vi "Leak check Protokoll_Kopf.vi"(11 "Externer Fehler":bool) -> ()   [LabVIEW 2020, in "EPA 1065.lvlib" / "Dichtheitstest 1065-345.lvlib"]
uses:
  Dichtheitstest 1065-345.lvlib
  Aktion Protokolldaten_Leak check.ctl
  Sprachverwaltung/FGV Aktion Tabelle zerlegen.ctl
  Funktionstasten/Funktionstasten-Aktion.ctl
  Seiten/System Einstellungen V2/Aktioen FGV System Konstanten.ctl
  Aktion Leak Daten.ctl
  PDF_Interface/PDF Protokoll Standard Kopf Optionen.ctl
  Sprachverwaltung/Sprachverwaltung.lvlib
  Funktionstasten/Funktionstasten.lvlib
  Seiten/System Einstellungen V2/System Einstellungen V2.lvlib
  Linearisierung V2/Protokoll/Protokoll.lvlib
  PDF_Interface/PDF Interface.lvlib
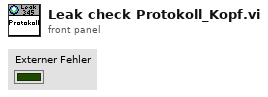
[diagram p1: front panel]
types:
  T1 = typedef "PDF Interface.lvlib/PDF Protokoll Standard Kopf Optionen.ctl" = cluster{"Analysator":bool, "FT-IR Rezept":bool, "Gasteiler":bool, "Gas Komponente":bool, "Gas Flasche":bool, "LIN Protokoll":bool, "Operator":bool}
  T2 = typedef "EPA 1065.lvlib/Dichtheitstest 1065-345.lvlib/Aktion Leak Daten.ctl" = enum16{"lesen", "laden", "speichern", "Volumen", "berechnen", "Leak check aktiv", "Leak Zustand", "Pfad", "Pfad speichern"}
  T3 = typedef "System Einstellungen V2.lvlib/Aktioen FGV System Konstanten.ctl" = enum16{"lesen", "laden", "speichern", "Sprache"}
  T4 = typedef "Funktionstasten.lvlib/Funktionstasten-Aktion.ctl" = enum16{"Initialisieren", "Zustand setzen", "Taste gedrückt", "Fehler speichern", "Lesen", "Manuell", "Remote", "Bitparallel", "Samplepoint", "Zeit Prüfen", "reset Umschalten"}
  T5 = typedef "Sprachverwaltung.lvlib/FGV Aktion Tabelle zerlegen.ctl" = enum16{"laden", "vereinzeln", "speichern"}
  T6 = typedef "EPA 1065.lvlib/Dichtheitstest 1065-345.lvlib/Aktion Protokolldaten_Leak check.ctl" = enum16{"lesen", "Zeitstempel", "Bearbeiter", "Daten", "Auswertung", "löschen"}
  T7 = typedef "EPA 1065.lvlib/Dichtheitstest 1065-345.lvlib/Leak Daten.ctl" = cluster{"Gesamtes Volumen":sgl, "p 1":sgl, "p 2":sgl, "T 1":sgl, "T 2":sgl, "t 1":timestamp, "t 2":timestamp, "Ergebnis mol/s":sgl, "Grenze mol/s":sgl, "Leak in %":sgl, "Ergebnis mbar":sgl, "Grenze mbar":sgl}
  T8 = cluster{"Modell":string, "ProjektNummer":string, "Software Version":string, "Seriennummer":string}
  T9 = typedef "EPA 1065.lvlib/Dichtheitstest 1065-345.lvlib/Gesamtvolumen.ctl" = cluster{"FAS":sgl, "d von HL zu VFS":sgl, "l von HL zu VFS":sgl, "VFS":sgl, "d von HL zu SP":sgl, "l von HL zu SP":sgl, "Heizleitung zum VFS":bool, "VFS a":bool, "Heizleitung zur Entnahmestelle":bool, "Gesamtes Volumen":sgl, "LeakValve":u16, "Einheit":enum16{"mol/s", "mbar"}}
  T10 = typedef "EPA 1065.lvlib/Dichtheitstest 1065-345.lvlib/Leak Protokoll Einstellungen.ctl" = cluster{"Bearbeiter:":string, "Pfad:":path, "Textname:":string, "Analysator":T11}
  T11 = typedef "System Einstellungen V2.lvlib/Analysatoren.ctl" = string
  T12 = typedef "String - Ausgabefeld.ctl" = string
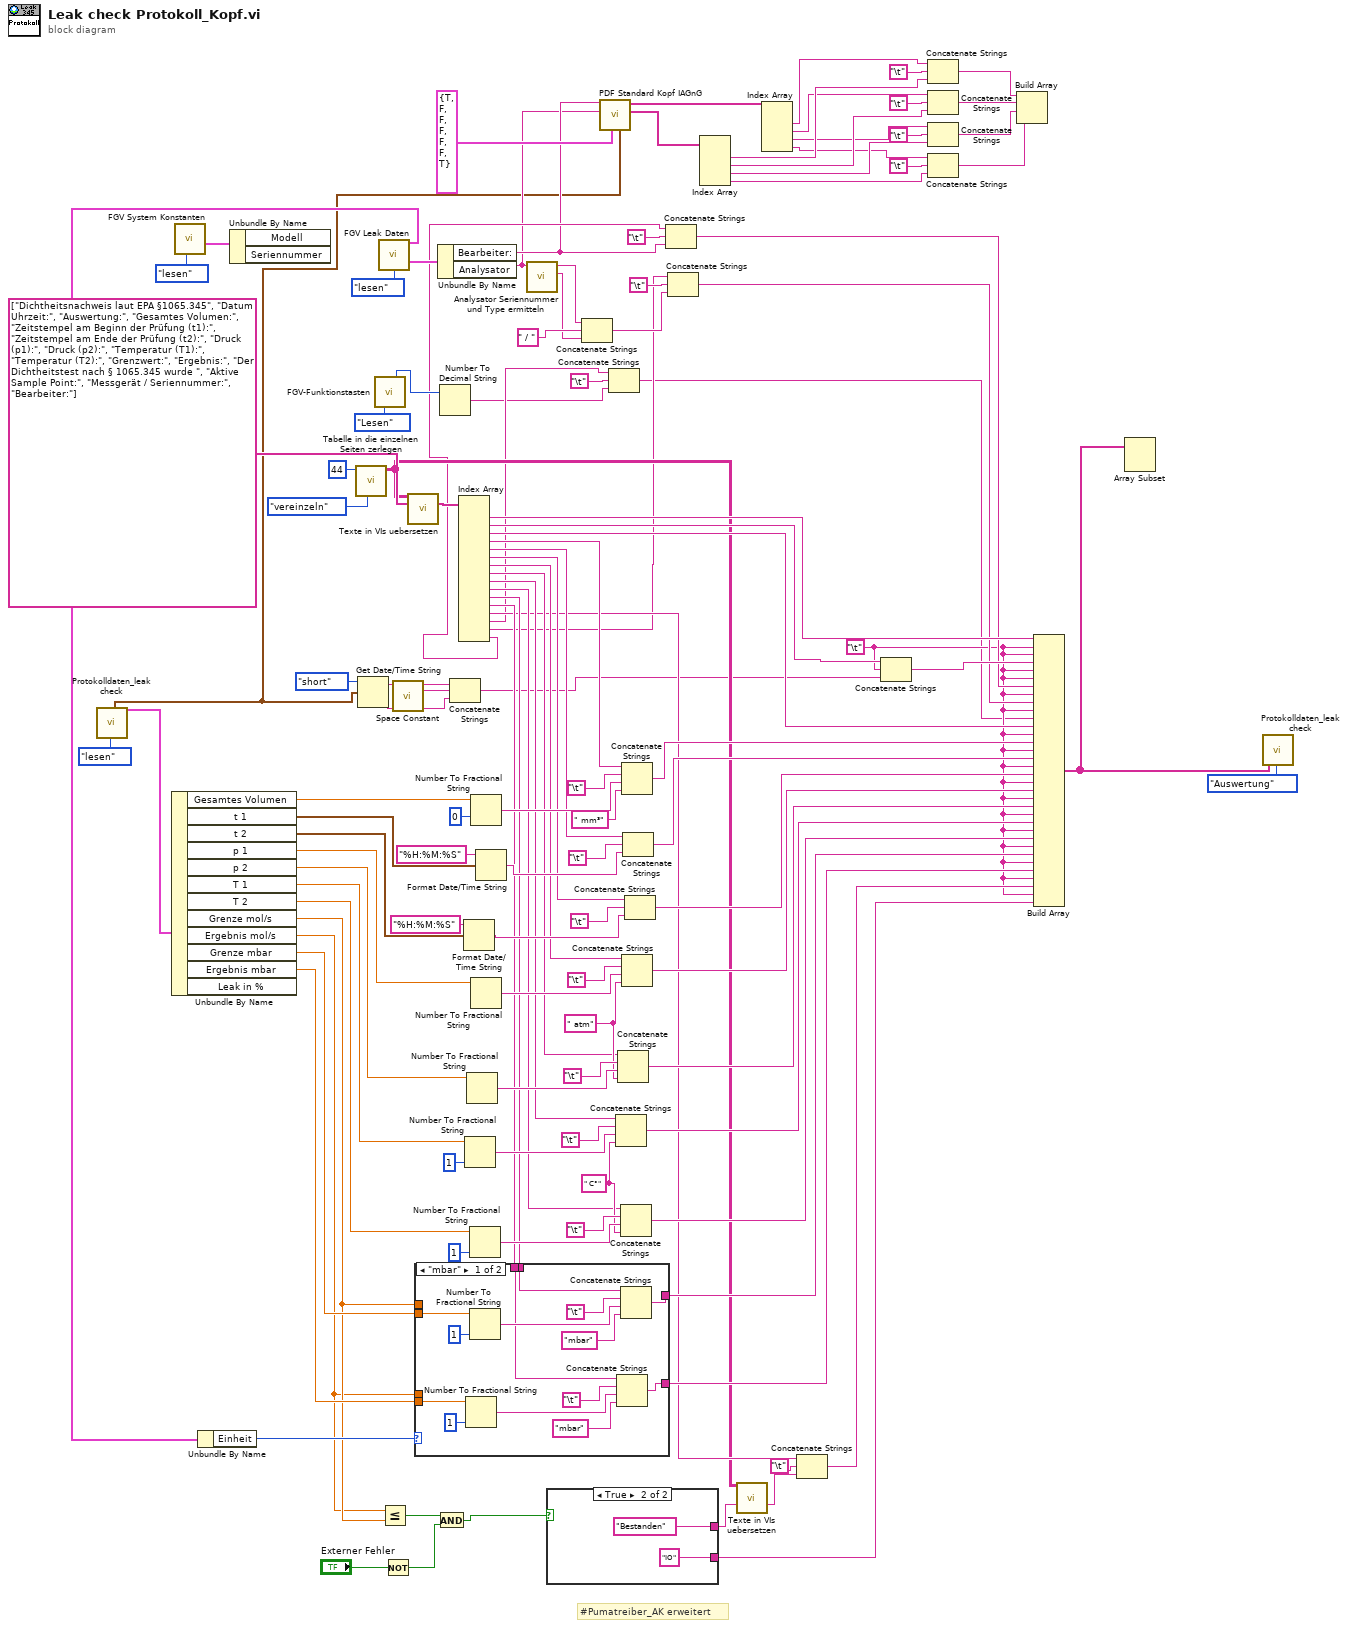
[diagram p0: block diagram]
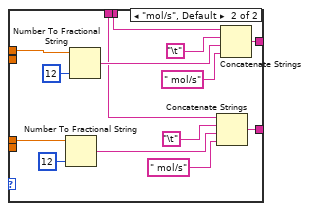
[diagram p2: hidden frame]
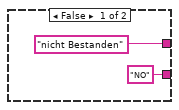
[diagram p3: hidden frame]
diagram:
  w42 = "\t"
  w99 = " C°"
  w100 = " atm"
  # "#Pumatreiber_AK erweitert"
  n1 = call "Protokolldaten_leak check.vi"("Aktion"=Aktion_Protokolldaten_Leak_check."lesen") -> ("Start"=w1:timestamp, "Daten"=w39:T7)  [unwired: 23 in, 2 out]
  n2 = Unbundle By Name(w39) -> ("Gesamtes Volumen"=w38:sgl, "t 1"=w37:timestamp, "t 2"=w36:timestamp, "p 1"=w35:sgl, "p 2"=w34:sgl, "T 1"=w33:sgl, "T 2"=w32:sgl, "Grenze mol/s"=w27:sgl, "Ergebnis mol/s"=w26:sgl, "Grenze mbar"=w28:sgl, "Ergebnis mbar"=w29:sgl)  [unwired: 1 out]
  n3 = call "FGV System Konstanten.vi"("Aktionen"=Aktioen_FGV_System_Konstanten."lesen") -> ("Cluster out"=w53:T8)  [unwired: 6 in, 4 out]
  n4 = Unbundle By Name(w53) -> ()  [unwired: 2 out]
  n5 = call "Tabelle in die einzelnen Seiten zerlegen.vi"("Aktion"=FGV_Aktion_Tabelle_zerlegen."vereinzeln", "Index (Seite)"=44) -> ("Sprachliste"=w64:string[][])  [unwired: 7 in, 2 out]
  n6 = Get Date/Time String(date format (0)=enum16{"short", "long", "abbreviated"}."short" ("Datumsformat (0)"), seconds (now)=w1) -> (date string=w122:string, time string=w120:string)  [unwired: 1 in]
  n7 = call "FGV-Funktionstasten.vi"("Aktion"=Funktionstasten-Aktion."Lesen") -> ("Samplepoint"=w56:u16)  [unwired: 7 in, 7 out]
  n8 = call "FGV Leak Daten.vi"("Aktion"=Aktion_Leak_Daten."lesen") -> ("Gesamtvolumen"=w31:T9, "Leak Protokoll"=w47:T10)  [unwired: 10 in, 3 out]
  n9 = Unbundle By Name(w31) -> ("Einheit"=w30:enum16{"mol/s", "mbar"})
  n10 = Less Or Equal?(x=w26, y=w27) -> (x <= y?=w84:bool)
  n11 = Not(x="Externer Fehler") -> (.not. x?=w83:bool)
  n12 = call <vilib>:"Space Constant.vi"() -> ("String"=w121:string)
  n13 = call "Texte in VIs uebersetzen.vi"("Sprachliste"=w64, "String-Array zum Übersetzen"=string[] ["Dichtheitsnachweis laut EPA §1065.345", "Datum Uhrzeit:", "Auswertung:", "Gesamtes Volumen:", "Zeitstempel am Beginn der Prüfung (t1):", "Zeitstempel am Ende der Prüfung (t2):", "Druck (p1):", "Druck (p2):", "Temperatur (T1):", "Temperatur (T2):", "Grenzwert:", "Ergebnis:", "Der Dichtheitstest nach § 1065.345 wurde ", "Aktive Sample Point:", "Messgerät / Seriennummer:", "Bearbeiter:"]) -> ("String-Array zum Übersetzen"=w80:string[])  [unwired: 9 in, 4 out]
  n14 = And(x=w84, y=w83) -> (x .and. y?=w86:bool)
  n15 = Unbundle By Name(w47) -> ("Bearbeiter:"=w22:string, "Analysator"=w21:T11)
  n16 = Number To Decimal String(number=w56) -> (decimal integer string=w55:string)  [unwired: 1 in]
  n17 = Concatenate Strings(w122, w121, w120) -> (w60:string)
  n18 = Index Array(array=w80) -> (element #1=w79:string, element #2=w78:string, element #3=w77:string, element #4=w76:string, element #5=w75:string, element #6=w74:string, element #7=w73:string, element #8=w72:string, element #9=w71:string, element #10=w70:string, element #11=w69:string, element #12=w68:string, element #13=w67:string, element #14=w57:string, element #15=w49:string, element #16=w45:string)  [unwired: 16 in]
  n19 = case shown="\"mbar\"" w30 {
    tunnel: [w132 w146] -> w98
    tunnel: [w131 w145] -> w97
    tunnel: w69 -> [w128 w142]
    tunnel: w68 -> [w127 w141]
    tunnel: w27 -> [_ w140]
    tunnel: w26 -> [_ w139]
    tunnel: w28 -> [w126 _]
    tunnel: w29 -> [w125 _]
    frame "mbar" {
      n20 = Number To Fractional String(number=w125, precision (6)=i16 1 ("Genauigkeit (6)")) -> (F-format string=w133:string)  [unwired: 2 in]
      n21 = Number To Fractional String(number=w126, precision (6)=i16 1 ("Genauigkeit (6)")) -> (F-format string=w138:string)  [unwired: 2 in]
      n22 = Concatenate Strings(w127, "\t", w133, "mbar") -> (w131:string)
      n23 = Concatenate Strings(w128, "\t", w138, "mbar") -> (w132:string)
    }
    frame "mol/s", Default {
      n24 = Number To Fractional String(number=w139, precision (6)=i16 12 ("Genauigkeit (6)")) -> (F-format string=w147:string)  [unwired: 2 in]
      n25 = Number To Fractional String(number=w140, precision (6)=i16 12 ("Genauigkeit (6)")) -> (F-format string=w152:string)  [unwired: 2 in]
      n26 = Concatenate Strings(w141, "\t", w147, " mol/s") -> (w145:string)
      n27 = Concatenate Strings(w142, "\t", w152, " mol/s") -> (w146:string)
    }
  }
  n28 = Format Date/Time String(time format string (%c)="%H:%M:%S" ("Zeitformatierungs-String (%c)"), seconds (now)=w36) -> (date/time string=w88:string)  [unwired: 1 in]
  n29 = Number To Fractional String(number=w33, precision (6)=i16 1 ("Genauigkeit (6)")) -> (F-format string=w108:string)  [unwired: 2 in]
  n30 = Number To Fractional String(number=w34) -> (F-format string=w109:string)  [unwired: 3 in]
  n31 = Number To Fractional String(number=w32, precision (6)=i16 1 ("Genauigkeit (6)")) -> (F-format string=w105:string)  [unwired: 2 in]
  n32 = Number To Fractional String(number=w38, precision (6)=i16 0 ("Genauigkeit (6)")) -> (F-format string=w118:string)  [unwired: 2 in]
  n33 = Number To Fractional String(number=w35) -> (F-format string=w116:string)  [unwired: 3 in]
  n34 = Format Date/Time String(time format string (%c)="%H:%M:%S" ("Zeitformatierungs-String (%c)"), seconds (now)=w37) -> (date/time string=w90:string)  [unwired: 1 in]
  n35 = call "Analysator Seriennummer und Type ermitteln.vi"("Analysator"=w21) -> ("Type"=w24:string, "Name für Protokoll"=w25:string)  [unwired: 8 in, 1 out]
  n36 = case shown="True" w86 {
    tunnel: ["nicht Bestanden" ("Element") "Bestanden" ("Element")] -> w66
    tunnel: ["NO" ("Element") "IO" ("Element")] -> w40
    frame False {
    }
    frame True {
    }
  }
  n37 = Concatenate Strings(w25, " / ", w24) -> (w50:string)
  n38 = call "PDF Standard Kopf IAGnG.vi"("Zeitstempel"=w1, "Oprtionen Cluster"=T1 {"Analysator"=TRUE, "FT-IR Rezept"=FALSE, "Gasteiler"=FALSE, "Gas Komponente"=FALSE, "Gas Flasche"=FALSE, "LIN Protokoll"=FALSE, "Operator"=TRUE}, "Analysator"=w21, "Bearbeiter/in"=w22) -> ("Header Values"=w19:T12[], "Header Labels"=w20:string[])  [unwired: 4 in, 2 out]
  n39 = Concatenate Strings(w57, "\t", w55) -> (w41:string)
  n40 = Concatenate Strings(w71, "\t", w108, w99) -> (w102:string)
  n41 = Concatenate Strings(w72, "\t", w109, w100) -> (w103:string)
  n42 = Concatenate Strings(w70, "\t", w105, w99) -> (w101:string)
  n43 = Concatenate Strings(w76, "\t", w118, " mm³") -> (w117:string)
  n44 = Concatenate Strings(w73, "\t", w116, w100) -> (w104:string)
  n45 = Concatenate Strings(w75, "\t", w90) -> (w113:string)
  n46 = Concatenate Strings(w74, "\t", w88) -> (w111:string)
  n47 = Concatenate Strings(w45, "\t", w22) -> (w44:string)
  n48 = Concatenate Strings(w49, "\t", w50) -> (w43:string)
  n49 = Index Array(array=w19) -> (element #1=w13:T12, element #2=w11:T12, element #3=w9:T12, element #4=w7:T12)  [unwired: 4 in]
  n50 = call "Texte in VIs uebersetzen.vi"("Sprachliste"=w64, "String zum Übersetzen"=w66) -> ("String zum Übersetzen"=w65:string)  [unwired: 9 in, 4 out]
  n51 = Index Array(array=w20) -> (element #1=w14:string, element #2=w12:string, element #3=w10:string, element #4=w8:string)  [unwired: 4 in]
  n52 = Concatenate Strings(w67, "\t", w65) -> (w96:string)
  n53 = Concatenate Strings(w78, w42, w60) -> (w61:string)
  n54 = Concatenate Strings(w14, "\t", w13) -> (w5:string)
  n55 = Concatenate Strings(w12, "\t", w11) -> (w4:string)
  n56 = Concatenate Strings(w10, "\t", w9) -> (w3:string)
  n57 = Concatenate Strings(w8, "\t", w7) -> (w2:string)
  n58 = Build Array(w5, w4, w3, w2) -> ()  [unwired: 1 out]
  n59 = Build Array(w79, w42, w42, w61, w42, w42, w44, w42, w43, w42, w41, w77, w42, w117, w42, w113, w42, w111, w42, w104, w42, w103, w42, w102, w42, w101, w42, w98, w42, w97, w42, w96, w42, w40) -> (w6:string[])
  n60 = Array Subset(array=w6) -> ()  [unwired: 2 in, 1 out]
  n61 = call "Protokolldaten_leak check.vi"("Auswertung"=w6, "Aktion"=Aktion_Protokolldaten_Leak_check."Auswertung") -> ()  [unwired: 22 in, 4 out]
